vi "ReadToFMulti.vi"(8 "error in":errorcluster, 9 "VL6180 Resources":T1[](array[typedef]) {"I2C Slave Address" format="%02x"}, 11 "LINX Resource in":T2) -> (0 "error out":errorcluster, 1 "VL Configs":T1[](array[typedef]) {"I2C Slave Address" format="%02x"}, 2 "Distance Readings":u8[](array[numeric]), 3 "LINX Resource out":T2)   [LabVIEW 2014]
uses:
  Sensors/Time of Flight - VL6180/VL6180 Resource.ctl
  <vilib>/MakerHub/LINX/Private/Type Defs/LINX Ref.ctl
  <vilib>/MakerHub/LINX/Private/Type Defs/Platform.ctl
  <vilib>/MakerHub/LINX/Private/Type Defs/Interface.ctl
  <vilib>/MakerHub/LINX/Private/Device/Type Defs/LINX Device Config.ctl
  <vilib>/MakerHub/LINX/Private/Device/Type Defs/TCP Config.ctl
  <vilib>/MakerHub/LINX/Private/Device/Type Defs/Channels.ctl
  <vilib>/MakerHub/LINX/LMH-LINX.lvlib
  <vilib>/MakerHub/LINX/Private/Device/Device.lvlib
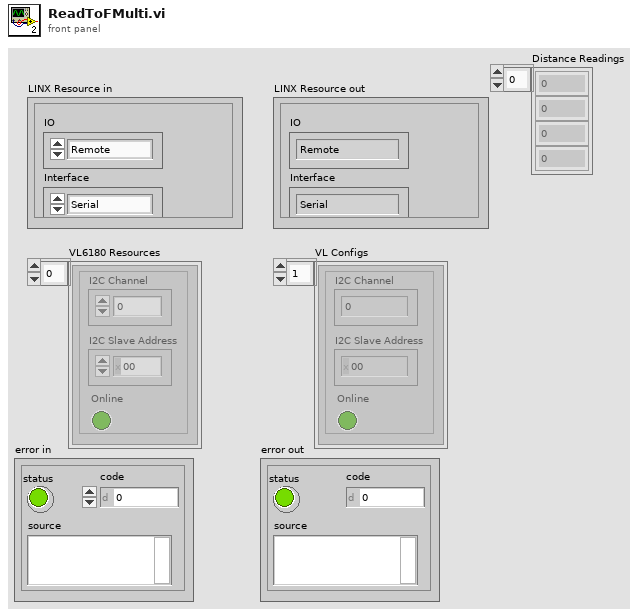
[diagram p1: front panel]
types:
  T1 = typedef "VL6180 Resource.ctl" = cluster{"I2C Channel":u8, "I2C Slave Address":u8, "Online":bool}
  T2 = typedef "LMH-LINX.lvlib/LINX Ref.ctl" = cluster{"IO":T3, "Interface":T4, "LINX Device Config":T5}
  T3 = typedef "LMH-LINX.lvlib/Platform.ctl" = enum16{"Remote", "Local"}
  T4 = typedef "LMH-LINX.lvlib/Interface.ctl" = enum16{"Serial", "TCP"}
  T5 = typedef "LMH-LINX.lvlib/Device.lvlib/LINX Device Config.ctl" = cluster{"Interface":T4, "COM Port":refnum<visa-resource-name>, "TCP Configuration":T6, "Device Family":u8, "Device ID":u8, "Device Name":string, "TCP Ref":refnum<k5>, "Channels":T7}
  T6 = typedef "LMH-LINX.lvlib/Device.lvlib/TCP Config.ctl" = cluster{"IP Address":string, "Port":u16}
  T7 = typedef "LMH-LINX.lvlib/Channels.ctl" = cluster{"DI":u8[], "DO":u8[], "AI":u8[], "AO":u8[], "PWM":u8[], "QE":u8[], "UART":u8[], "I2C 2":u8[], "SPI":u8[], "CAN":u8[], "Servo":u8[], "AI Ref (V)":dbl, "AI Resolution (Bits)":u8, "AO Ref (V)":dbl, "AO Resolution (Bits)":u8}
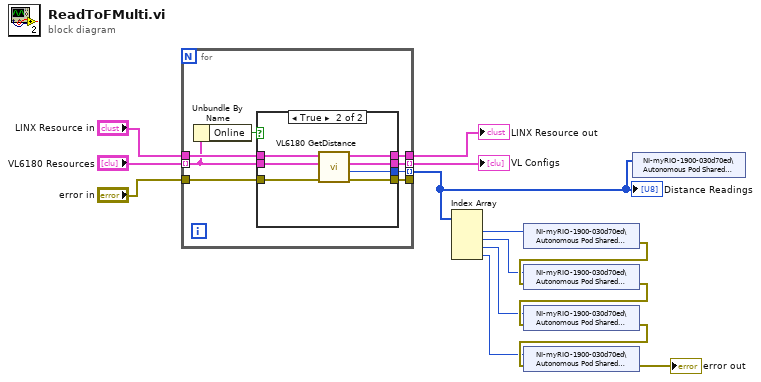
[diagram p0: block diagram]
diagram:
  n1 = for {
    tunnel: "VL6180 Resources" -> [w16] mode=indexing
    tunnel: "LINX Resource in" -> [w22]
    tunnel: "error in" -> [w19]
    tunnel: [w21] -> w13
    tunnel: [w20] -> w14 mode=indexing
    tunnel: [w18] -> _
    tunnel: [w17] -> w1 mode=indexing
    n2 = Unbundle By Name(w16) -> ("Online"=w15:bool)
    n3 = case shown="True" w15 {
      tunnel: w22 -> [w25 w32]
      tunnel: w16 -> [w24 w31]
      tunnel: [w25 w30] -> w21
      tunnel: [w24 w29] -> w20
      tunnel: w19 -> [w23 w28]
      tunnel: [w23 w27] -> w18
      tunnel: [_ w26] -> w17
      frame False {
      }
      frame True {
        n4 = call "VL6180 GetDistance.vi"("error in (no error)"=w28, "VL6180 Resource in"=w31, "LINX Resource"=w32) -> ("error out"=w27:errorcluster, "Distance (mm)"=w26:u8, "VL6180 Resource out"=w29:T1, "LINX Resource"=w30:T2)  [unwired: 4 in, 1 out]
      }
    }
  }
  "VL Configs" <- w14
  "LINX Resource out" <- w13
  "Distance Readings" <- w1
  n5 = Index Array(array=w1) -> (element #1=w9:u8, element #2=w4:u8, element #3=w2:u8, element #4=w3:u8)  [unwired: 4 in]
  n6 = shared-variable "NI-myRIO-1900-030d70ed\\Autonomous Pod Shared Variables.lvlib\\ToF1Distance"(w9) -> (error out=w8:errorcluster)  [unwired: 1 in]
  n7 = shared-variable "NI-myRIO-1900-030d70ed\\Autonomous Pod Shared Variables.lvlib\\ToF2Distance"(w4, error in=w8) -> (error out=w7:errorcluster)
  n8 = shared-variable "NI-myRIO-1900-030d70ed\\Autonomous Pod Shared Variables.lvlib\\ToF3Distance"(w2, error in=w7) -> (error out=w6:errorcluster)
  n9 = shared-variable "NI-myRIO-1900-030d70ed\\Autonomous Pod Shared Variables.lvlib\\ToF4Distance"(w3, error in=w6) -> (error out=→"error out":errorcluster)
  n10 = shared-variable "NI-myRIO-1900-030d70ed\\Autonomous Pod Shared Variables.lvlib\\ToFReadings"(w1) -> ()  [unwired: 1 in, 1 out]
